vi "Check Key Exists.vi"(7 "Crypto Provider":T1, 8 "error in (no error)":errorcluster, 11 "Key Name":string) -> (0 "error out":errorcluster, 3 "Key Exists?":bool)   [LabVIEW 2021, in "dotNET Crypto Key Management.lvlib"]
uses:
  dotNET Crypto Key Management.lvlib
  CNG Provider Type.ctl
  System.Core
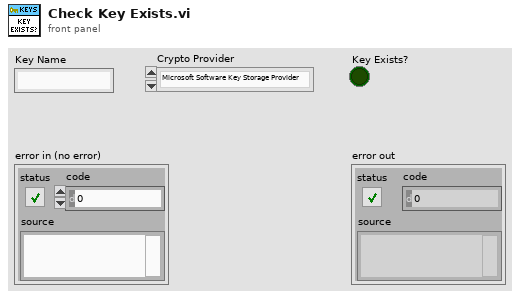
[diagram p1: front panel]
types:
  T1 = typedef "dotNET Crypto Key Management.lvlib/CNG Provider Type.ctl" = enum16{"Microsoft Software Key Storage Provider", "Microsoft Platform Crypto Provider"}
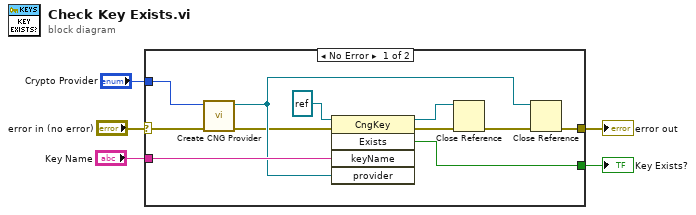
[diagram p0: block diagram]
diagram:
  n1 = case shown="No Error" "error in (no error)" {
    selector: "error in (no error)" -> [w7 w17]
    tunnel: "Key Name" -> [w14 _]
    tunnel: [w13 _] -> w4
    tunnel: "Crypto Provider" -> [w11 _]
    tunnel: [w9 w17] -> w2
    frame No Error {
      n2 = call "Create CNG Provider.vi"("error in (no error)"=w7, "Crypto Provider"=w11) -> ("error out"=w6:errorcluster, "CngProvider"=w8:refnum<k24>)  [unwired: 8 in]
      n3 = invoke class="CngKey" method="Exists"(reference=refnum<k24> refnum, error in=w6, "keyName"=w14, "provider"=w8) -> (reference out=w16:refnum<k24>, error out=w15:errorcluster, "Exists"=w13:bool)  [unwired: 1 in, 2 out]
      n4 = Close Reference(reference=w16, error in (no error)=w15) -> (error out=w10:errorcluster)
      n5 = Close Reference(reference=w8, error in (no error)=w10) -> (error out=w9:errorcluster)
    }
    frame Error {
    }
  }
  "error out" <- w2
  "Key Exists?" <- w4
